vi "Message UI.vi"(11 "Message Update":refnum<queue>) -> ()   [LabVIEW 2022 SP3, in "FlexBlocks Support.lvlib"]
uses:
  FlexBlocks Support.lvlib
panel:
  in  "Initial Message":string
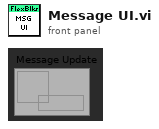
[diagram p1: front panel]
types:
  T1 = enum32{"Invalid", "Standard", "Closed", "Hidden", "Minimized", "Maximized"}
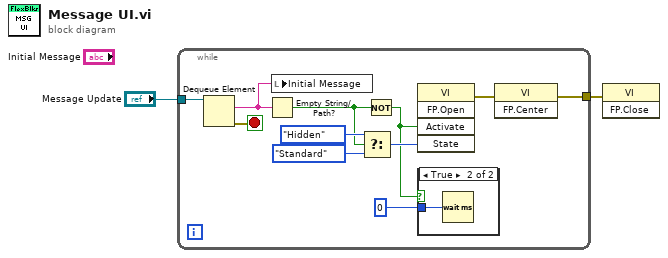
[diagram p0: block diagram]
diagram:
  n1 = while {
    tunnel: [w3] -> w2
    tunnel: "Message Update" -> [w9]
    stop <- w8 stop-if-true
    n2 = Dequeue Element(queue=w9) -> (element=w7:string, error out=w8:errorcluster)  [unwired: 2 in, 2 out]
    n3 = Empty String/Path?(string/path=w7) -> (empty?=w10:bool)
    n4 = local write "Initial Message"(w7) -> ()
    n5 = Select(t=T1."Hidden" ("State"), s=w10, f=T1."Standard" ("State")) -> (s? t:f=w11:T1)
    n6 = Not(x=w10) -> (.not. x?=w6:bool)
    n7 = invoke class="VI" method="FP.Open"("Activate"=w6, "State"=w11) -> (error out=w4:errorcluster)  [unwired: 3 in, 4 out]
    n8 = case shown="True" w6 {
      tunnel: u32 0 ("milliseconds to wait") -> [_ w14]
      frame False {
      }
      frame True {
        n9 = Wait (ms)(milliseconds to wait=w14) -> ()  [unwired: 1 out]
      }
    }
    n10 = invoke class="VI" method="FP.Center"(error in=w4) -> (error out=w3:errorcluster)  [unwired: 2 in, 2 out]
  }
  n11 = invoke class="VI" method="FP.Close"(error in=w2) -> ()  [unwired: 2 in, 3 out]
